vi "__GetDMM_34401A_plc.vi"(5 "DMM設定A":T1={"間隔"=1.0, "サンプルデータ数"=500, "Voltage Range"=enum."1 V", "Factor"=1.0, "単位"=1, " 電源周波数(Hz)"=50.0} {"単位" items=["Sec", "PLC"]; "サンプルデータ数" min=1 max=1000000 step=1}) -> (0 "電圧":dbl[](array[numeric]) format="%#_9g", 1 "時間":dbl[](array[numeric])=[0.0, 0.02, 0.04, 0.06, 0.08, 0.1, 0.12, 0.14, 0.16, 0.18, 0.2, 0.22, 0.24, 0.26, 0.28, 0.3, 0.32, 0.34, 0.36, 0.38, 0.4, 0.42, 0.44, 0.46, 0.48, 0.5, 0.52, 0.54, 0.56, 0.58, 0.6, 0.62, 0.64, 0.66, 0.68, 0.7000000000000001, 0.72, 0.74, 0.76, 0.78, 0.8, 0.8200000000000001, 0.84, 0.86, 0.88, 0.9, 0.92, 0.9400000000000001, 0.96, 0.98, 1.0, 1.02, 1.04, 1.06, 1.08, 1.1, 1.12, 1.1400000000000001, 1.16, 1.18, 1.2, 1.22, 1.24, 1.26, 1.28, 1.3, 1.32, 1.34, 1.36, 1.3800000000000001, 1.4000000000000001, 1.42, 1.44, 1.46, 1.48, 1.5, 1.52, 1.54, 1.56, 1.58, 1.6, 1.62, 1.6400000000000001, 1.6600000000000001, 1.68, 1.7, 1.72, 1.74, 1.76, 1.78, 1.8, 1.82, 1.84, 1.86, 1.8800000000000001, 1.9000000000000001, 1.92, 1.94, 1.96, 1.98, 2.0, 2.02, 2.04, 2.06, 2.08, 2.1, 2.12, 2.14, 2.16, 2.18, 2.2, 2.22, 2.24, 2.2600000000000002, 2.2800000000000002, 2.3000000000000003, 2.32, 2.34, 2.36, 2.38, 2.4, 2.42, 2.44, 2.46, 2.48, 2.5, 2.52, 2.54, 2.56, 2.58, 2.6, 2.62, 2.64, 2.66, 2.68, 2.7, 2.72, 2.74, 2.7600000000000002, 2.7800000000000002, 2.8000000000000003, 2.82, 2.84, 2.86, 2.88, 2.9, 2.92, 2.94, 2.96, 2.98, 3.0, 3.02, 3.04, 3.06, 3.08, 3.1, 3.12, 3.14, 3.16, 3.18, 3.2, 3.22, 3.24, 3.2600000000000002, 3.2800000000000002, 3.3000000000000003, 3.3200000000000003, 3.34, 3.36, 3.38, 3.4, 3.42, 3.44, 3.46, 3.48, 3.5, 3.52, 3.54, 3.56, 3.58, 3.6, 3.62, 3.64, 3.66, 3.68, 3.7, 3.72, 3.74, 3.7600000000000002, 3.7800000000000002, 3.8000000000000003, 3.8200000000000003, 3.84, 3.86, 3.88, 3.9, 3.92, 3.94, 3.96, 3.98, 4.0, 4.0200000000000005, 4.04, 4.0600000000000005, 4.08, 4.1, 4.12, 4.14, 4.16, 4.18, 4.2, 4.22, 4.24, 4.26, 4.28, 4.3, 4.32, 4.34, 4.36, 4.38, 4.4, 4.42, 4.44, 4.46, 4.48, 4.5, 4.5200000000000005, 4.54, 4.5600000000000005, 4.58, 4.6000000000000005, 4.62, 4.64, 4.66, 4.68, 4.7, 4.72, 4.74, 4.76, 4.78, 4.8, 4.82, 4.84, 4.86, 4.88, 4.9, 4.92, 4.94, 4.96, 4.98, 5.0, 5.0200000000000005, 5.04, 5.0600000000000005, 5.08, 5.1000000000000005, 5.12, 5.14, 5.16, 5.18, 5.2, 5.22, 5.24, 5.26, 5.28, 5.3, 5.32, 5.34, 5.36, 5.38, 5.4, 5.42, 5.44, 5.46, 5.48, 5.5, 5.5200000000000005, 5.54, 5.5600000000000005, 5.58, 5.6000000000000005, 5.62, 5.64, 5.66, 5.68, 5.7, 5.72, 5.74, 5.76, 5.78, 5.8, 5.82, 5.84, 5.86, 5.88, 5.9, 5.92, 5.94, 5.96, 5.98, 6.0, 6.0200000000000005, 6.04, 6.0600000000000005, 6.08, 6.1000000000000005, 6.12, 6.140000000000001, 6.16, 6.18, 6.2, 6.22, 6.24, 6.26, 6.28, 6.3, 6.32, 6.34, 6.36, 6.38, 6.4, 6.42, 6.44, 6.46, 6.48, 6.5, 6.5200000000000005, 6.54, 6.5600000000000005, 6.58, 6.6000000000000005, 6.62, 6.640000000000001, 6.66, 6.68, 6.7, 6.72, 6.74, 6.76, 6.78, 6.8, 6.82, 6.84, 6.86, 6.88, 6.9, 6.92, 6.94, 6.96, 6.98, 7.0, 7.0200000000000005, 7.04, 7.0600000000000005, 7.08, 7.1000000000000005, 7.12, 7.140000000000001, 7.16, 7.18, 7.2, 7.22, 7.24, 7.26, 7.28, 7.3, 7.32, 7.34, 7.36, 7.38, 7.4, 7.42, 7.44, 7.46, 7.48, 7.5, 7.5200000000000005, 7.54, 7.5600000000000005, 7.58, 7.6000000000000005, 7.62, 7.640000000000001, 7.66, 7.68, 7.7, 7.72, 7.74, 7.76, 7.78, 7.8, 7.82, 7.84, 7.86, 7.88, 7.9, 7.92, 7.94, 7.96, 7.98, 8.0, 8.02, 8.040000000000001, 8.06, 8.08, 8.1, 8.120000000000001, 8.14, 8.16, 8.18, 8.2, 8.22, 8.24, 8.26, 8.28, 8.3, 8.32, 8.34, 8.36, 8.38, 8.4, 8.42, 8.44, 8.46, 8.48, 8.5, 8.52, 8.540000000000001, 8.56, 8.58, 8.6, 8.620000000000001, 8.64, 8.66, 8.68, 8.700000000000001, 8.72, 8.74, 8.76, 8.78, 8.8, 8.82, 8.84, 8.86, 8.88, 8.9, 8.92, 8.94, 8.96, 8.98, 9.0, 9.02, 9.040000000000001, 9.06, 9.08, 9.1, 9.120000000000001, 9.14, 9.16, 9.18, 9.200000000000001, 9.22, 9.24, 9.26, 9.28, 9.3, 9.32, 9.34, 9.36, 9.38, 9.4, 9.42, 9.44, 9.46, 9.48, 9.5, 9.52, 9.540000000000001, 9.56, 9.58, 9.6, 9.620000000000001, 9.64, 9.66, 9.68, 9.700000000000001, 9.72, 9.74, 9.76, 9.78, 9.8, 9.82, 9.84, 9.86, 9.88, 9.9, 9.92, 9.94, 9.96, 9.98, 10.0, 10.02, 10.040000000000001, 10.06, 10.08, 10.1, 10.120000000000001, 10.14, 10.16, 10.18, 10.200000000000001, 10.22, 10.24, 10.26, 10.28, 10.3, 10.32, 10.34, 10.36, 10.38, 10.4, 10.42, 10.44, 10.46, 10.48, 10.5, 10.52, 10.540000000000001, 10.56, 10.58, 10.6, 10.620000000000001, 10.64, 10.66, 10.68, 10.700000000000001, 10.72, 10.74, 10.76, 10.78, 10.8, 10.82, 10.84, 10.86, 10.88, 10.9, 10.92, 10.94, 10.96, 10.98, 11.0, 11.02, 11.040000000000001, 11.06, 11.08, 11.1, 11.120000000000001, 11.14, 11.16, 11.18, 11.200000000000001, 11.22, 11.24, 11.26, 11.28, 11.3, 11.32, 11.34, 11.36, 11.38, 11.4, 11.42, 11.44, 11.46, 11.48, 11.5, 11.52, 11.540000000000001, 11.56, 11.58, 11.6, 11.620000000000001, 11.64, 11.66, 11.68, 11.700000000000001, 11.72, 11.74, 11.76, 11.78, 11.8, 11.82, 11.84, 11.86, 11.88, 11.9, 11.92, 11.94, 11.96, 11.98, 12.0, 12.02, 12.040000000000001, 12.06, 12.08, 12.1, 12.120000000000001, 12.14, 12.16, 12.18, 12.200000000000001, 12.22, 12.24, 12.26, 12.280000000000001, 12.3, 12.32, 12.34, 12.36, 12.38, 12.4, 12.42, 12.44, 12.46, 12.48, 12.5, 12.52, 12.540000000000001, 12.56, 12.58, 12.6, 12.620000000000001, 12.64, 12.66, 12.68, 12.700000000000001, 12.72, 12.74, 12.76, 12.780000000000001, 12.8, 12.82, 12.84, 12.86, 12.88, 12.9, 12.92, 12.94, 12.96, 12.98, 13.0, 13.02, 13.040000000000001, 13.06, 13.08, 13.1, 13.120000000000001, 13.14, 13.16, 13.18, 13.200000000000001, 13.22, 13.24, 13.26, 13.280000000000001, 13.3, 13.32, 13.34, 13.36, 13.38, 13.4, 13.42, 13.44, 13.46, 13.48, 13.5, 13.52, 13.540000000000001, 13.56, 13.58, 13.6, 13.620000000000001, 13.64, 13.66, 13.68, 13.700000000000001, 13.72, 13.74, 13.76, 13.780000000000001, 13.8, 13.82, 13.84, 13.86, 13.88, 13.9, 13.92, 13.94, 13.96, 13.98, 14.0, 14.02, 14.040000000000001, 14.06, 14.08, 14.1, 14.120000000000001, 14.14, 14.16, 14.18, 14.200000000000001, 14.22, 14.24, 14.26, 14.280000000000001, 14.3, 14.32, 14.34, 14.36, 14.38, 14.4, 14.42, 14.44, 14.46, 14.48, 14.5, 14.52, 14.540000000000001, 14.56, 14.58, 14.6, 14.620000000000001, 14.64, 14.66, 14.68, 14.700000000000001, 14.72, 14.74, 14.76, 14.780000000000001, 14.8, 14.82, 14.84, 14.86, 14.88, 14.9, 14.92, 14.94, 14.96, 14.98, 15.0, 15.02, 15.040000000000001, 15.06, 15.08, 15.1, 15.120000000000001, 15.14, 15.16, 15.18, 15.200000000000001, 15.22, 15.24, 15.26, 15.280000000000001, 15.3, 15.32, 15.34, 15.36, 15.38, 15.4, 15.42, 15.44, 15.46, 15.48, 15.5, 15.52, 15.540000000000001, 15.56, 15.58, 15.6, 15.620000000000001, 15.64, 15.66, 15.68, 15.700000000000001, 15.72, 15.74, 15.76, 15.780000000000001, 15.8, 15.82, 15.84, 15.860000000000001, 15.88, 15.9, 15.92, 15.94, 15.96, 15.98, 16.0, 16.02, 16.04, 16.06, 16.080000000000002, 16.1, 16.12, 16.14, 16.16, 16.18, 16.2, 16.22, 16.240000000000002, 16.26, 16.28, 16.3, 16.32, 16.34, 16.36, 16.38, 16.4, 16.42, 16.44, 16.46, 16.48, 16.5, 16.52, 16.54, 16.56, 16.580000000000002, 16.6, 16.62, 16.64, 16.66, 16.68, 16.7, 16.72, 16.740000000000002, 16.76, 16.78, 16.8, 16.82, 16.84, 16.86, 16.88, 16.9, 16.92, 16.94, 16.96, 16.98, 17.0, 17.02, 17.04, 17.06, 17.080000000000002, 17.1, 17.12, 17.14, 17.16, 17.18, 17.2, 17.22, 17.240000000000002, 17.26, 17.28, 17.3, 17.32, 17.34, 17.36, 17.38, 17.400000000000002, 17.42, 17.44, 17.46, 17.48, 17.5, 17.52, 17.54, 17.56, 17.580000000000002, 17.6, 17.62, 17.64, 17.66, 17.68, 17.7, 17.72, 17.740000000000002, 17.76, 17.78, 17.8, 17.82, 17.84, 17.86, 17.88, 17.900000000000002, 17.92, 17.94, 17.96, 17.98, 18.0, 18.02, 18.04, 18.06, 18.080000000000002, 18.1, 18.12, 18.14, 18.16, 18.18, 18.2, 18.22, 18.240000000000002, 18.26, 18.28, 18.3, 18.32, 18.34, 18.36, 18.38, 18.400000000000002, 18.42, 18.44, 18.46, 18.48, 18.5, 18.52, 18.54, 18.56, 18.580000000000002, 18.6, 18.62, 18.64, 18.66, 18.68, 18.7, 18.72, 18.740000000000002, 18.76, 18.78, 18.8, 18.82, 18.84, 18.86, 18.88, 18.900000000000002, 18.92, 18.94, 18.96, 18.98, 19.0, 19.02, 19.04, 19.06, 19.080000000000002, 19.1, 19.12, 19.14, 19.16, 19.18, 19.2, 19.22, 19.240000000000002, 19.26, 19.28, 19.3, 19.32, 19.34, 19.36, 19.38, 19.400000000000002, 19.42, 19.44, 19.46, 19.48, 19.5, 19.52, 19.54, 19.56, 19.580000000000002, 19.6, 19.62, 19.64, 19.66, 19.68, 19.7, 19.72, 19.740000000000002, 19.76, 19.78, 19.8, 19.82, 19.84, 19.86, 19.88, 19.900000000000002, 19.92, 19.94, 19.96, 19.98])   [LabVIEW 2017]
panel:
  in  "VOLT":dbl
  out "XYグラフ":cluster{"x":dbl[], dbl[]}(graph)
  in  "Instr.ID":string="22"
  out "文字列":string
  # "t_facotr\nPLC=1 =>1\nPLC=0.1 => 1.0135\nPLC=0.01 => 1.1321"
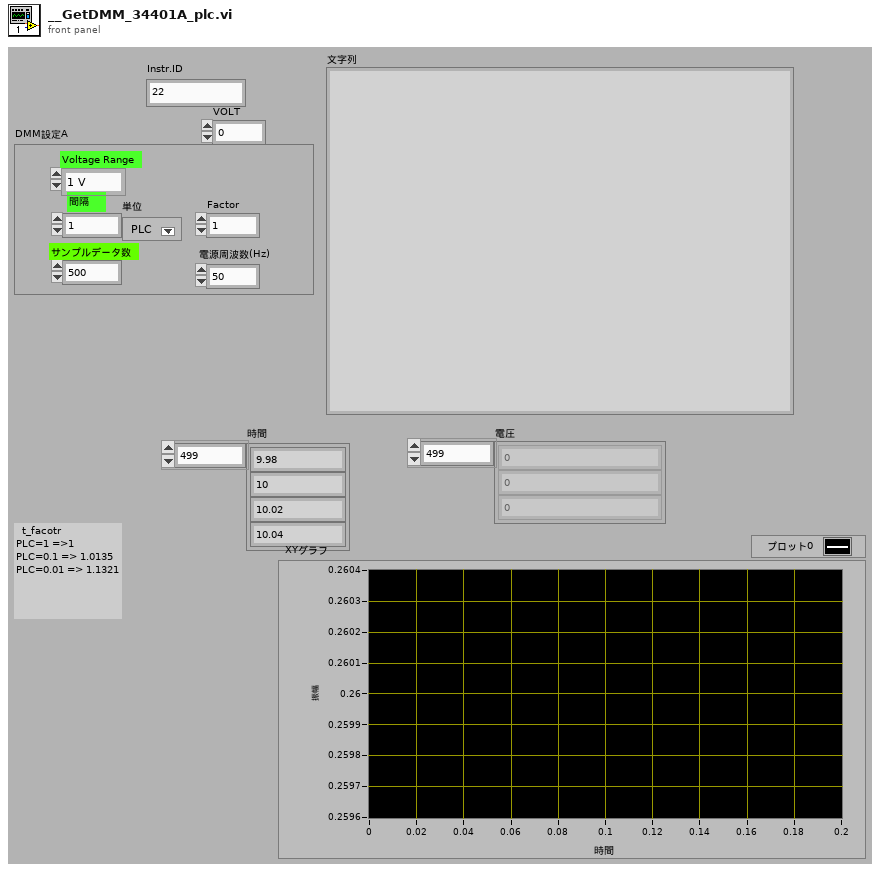
[diagram p1: front panel]
types:
  T1 = cluster{"間隔":dbl, "サンプルデータ数":i32, "Voltage Range":enum16{"100 mV", "1 V", "10 V", "100 V", "1000 V", "Auto", "Minimum", "Maximum"}, "Factor":dbl, "単位":u16, " 電源周波数(Hz)":dbl}
  T2 = enum16{"100 mV", "1 V", "10 V", "100 V", "1000 V", "Auto", "Minimum", "Maximum"}
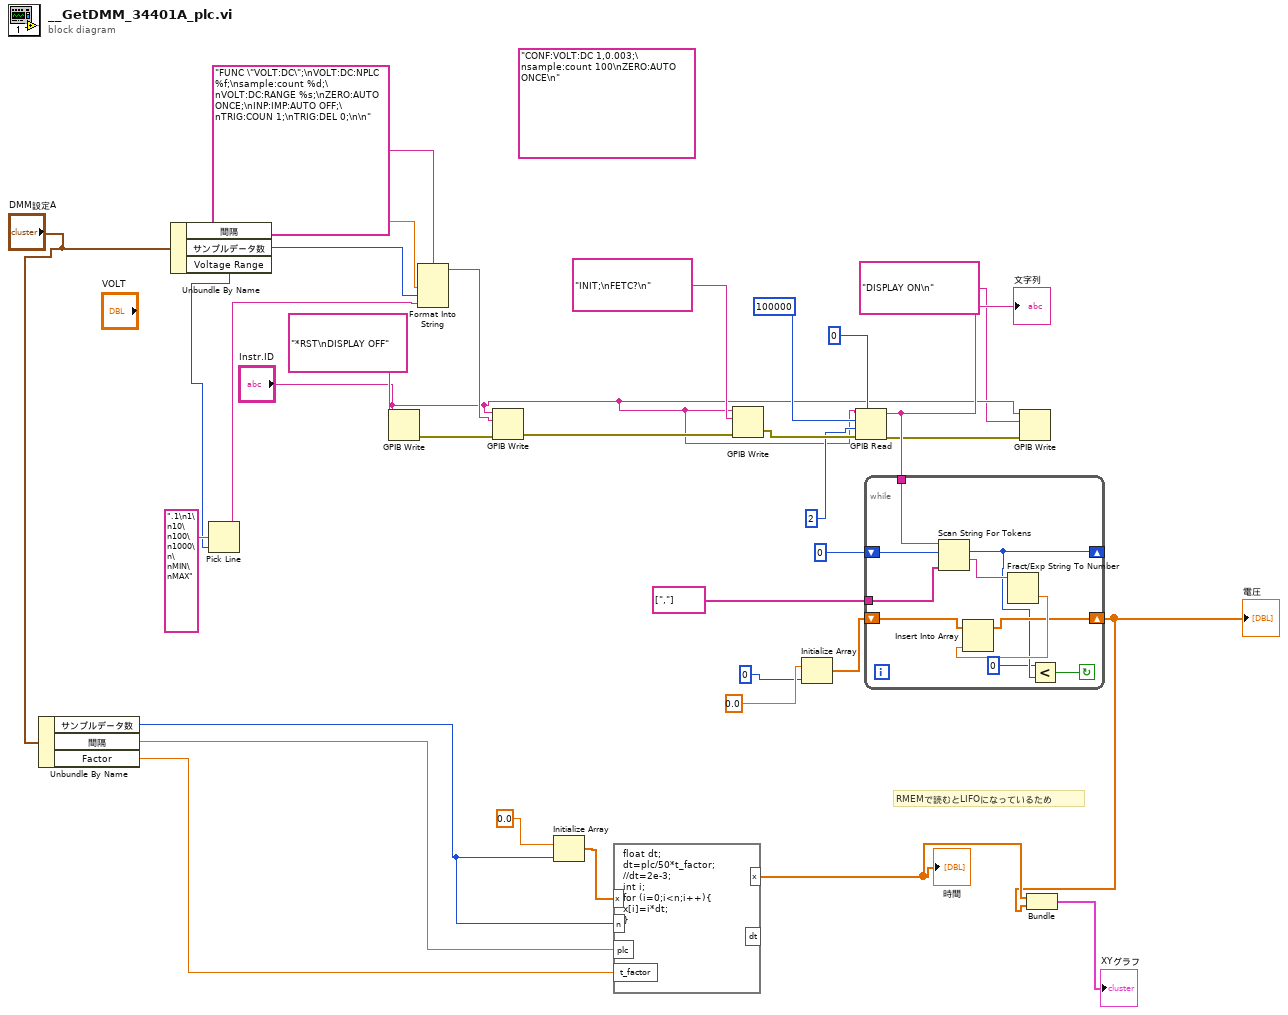
[diagram p0: block diagram]
diagram:
  (unwired) "CONF:VOLT:DC 1,0.003;\nsample:count 100\nZERO:AUTO ONCE\n"
  # "RMEMで読むとLIFOになっているため"
  n1 = Unbundle By Name("DMM設定A") -> ("サンプルデータ数"=w10:i32, "間隔"=w11:dbl, "Factor"=w14:dbl)
  n2 = Unbundle By Name("DMM設定A") -> ("間隔"=w18:dbl, "サンプルデータ数"=w17:i32, "Voltage Range"=w1:T2)
  n3 = Pick Line(multi-line string=".1\n1\n10\n100\n1000\n\nMIN\nMAX", line index=w1) -> (output string=w2:string)  [unwired: 1 in]
  n4 = GPIB Write(0:"Instr.ID", 1:"*RST\nDISPLAY OFF") -> (6:w31:errorcluster)  [unwired: 3 in, 1 out]
  n5 = Format Into String(format string="FUNC \"VOLT:DC\";\nVOLT:DC:NPLC %f;\nsample:count %d;\nVOLT:DC:RANGE %s;\nZERO:AUTO ONCE;\nINP:IMP:AUTO OFF;\nTRIG:COUN 1;\nTRIG:DEL 0;\n\n", w18, w17, w2) -> (resulting string=w7:string)  [unwired: 2 in, 1 out]
  n6 = GPIB Write(0:"Instr.ID", 1:w7, 3:w31) -> (6:w27:errorcluster)  [unwired: 2 in, 1 out]
  n7 = Initialize Array(0.0, w10) -> (w15:dbl[])
  n8 = formula code="float dt;\ndt=plc/50*t_factor;\n//dt=2e-3;\nint i;\nfor (i=0;i<n;i++){\nx[i]=i*dt;\n}"("x"=w15, "n"=w10, "plc"=w11, "t_factor"=w14) -> ("x"=w13:dbl[])  [unwired: 1 out]
  "時間" <- w13
  n9 = GPIB Write(0:"Instr.ID", 1:"INIT;\nFETC?\n", 3:w27) -> (6:w26:errorcluster)  [unwired: 2 in, 1 out]
  n10 = Initialize Array(0.0, 0) -> (w21:dbl[])
  n11 = GPIB Read(0:"Instr.ID", 1:100000, 2:2, 3:w26, 4:0) -> (5:w22:string, 7:w5:errorcluster)  [unwired: 1 out]
  "文字列" <- w22
  n12 = while {
    tunnel: string[] [","] -> [w43]
    shift-right: [w36] -> _
    shift-left: 0 -> [w42]
    shift-right: [w38] -> w8
    shift-left: w21 -> [w40]
    tunnel: w22 -> [w34]
    stop <- w37 continue-if-true
    n13 = Scan String For Tokens(6:w43, 8:w42, 9:w34) -> (1:w41:string, 2:w36:i32)  [unwired: 3 in, 2 out]
    n14 = Fract/Exp String To Number(string=w41) -> (number=w39:dbl)  [unwired: 3 in, 1 out]
    n15 = Insert Into Array(array=w40, new element=w39) -> (w38:dbl[])  [unwired: 1 in]
    n16 = Less?(x=0, y=w36) -> (x < y?=w37:bool)
  }
  "電圧" <- w8
  n17 = GPIB Write(0:"Instr.ID", 1:"DISPLAY ON\n", 3:w5) -> ()  [unwired: 2 in, 2 out]
  n18 = Bundle("x"=w13, w8) -> (→"XYグラフ":cluster{"x":dbl[], dbl[]})  [unwired: 1 in]
